vi "flushTank.vi"(8 "error in (no error)":errorcluster, 10 "Index":i32, 11 "Tank in":refnum<class "Tank.lvclass">) -> (0 "error out":errorcluster, 3 "Tank out":refnum<class "Tank.lvclass">)   [LabVIEW 2018, in "Tank.lvclass"]
uses:
  Tank.lvclass
  Tank.lvclass/Tank.ctl
  Sensor Class/Sensor.lvclass/Sensor.ctl
  Sensor Class/Sensor.lvclass
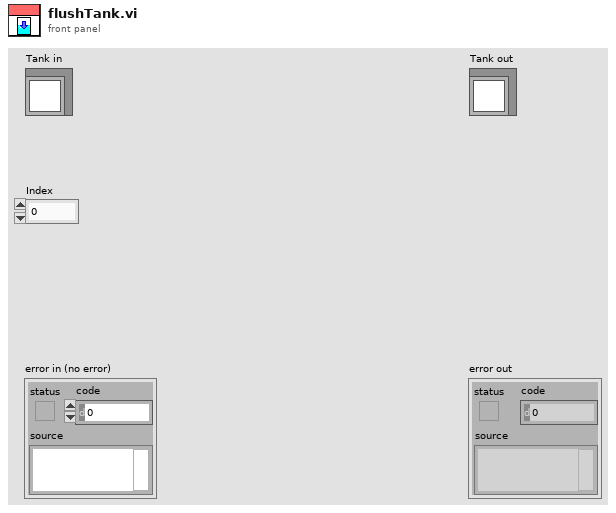
[diagram p1: front panel]
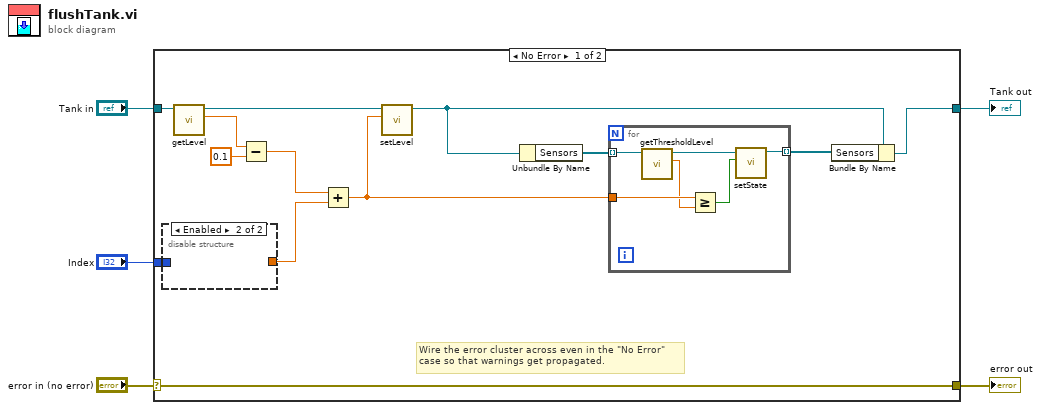
[diagram p0: block diagram]
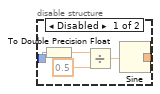
[diagram p2: hidden frame]
diagram:
  n1 = case shown="No Error" "error in (no error)" {
    selector: "error in (no error)" -> [w18 w31]
    tunnel: [w18 w31] -> w4
    tunnel: [w16 w30] -> w2
    tunnel: "Tank in" -> [w17 w30]
    tunnel: "Index" -> [w12 _]
    frame No Error {
      # "Wire the error cluster across even in the \"No Error\"\ncase so that warnings get propagated."
      n2 = disable-structure shown="Enabled" {
        disable-tunnel: [w23 _] -> w15
        disable-tunnel: w12 -> [w22 _]
        frame Disabled {
          n3 = To Double Precision Float(number=w22) -> (double precision float=w20:dbl)
          n4 = Divide(x=w20, y=0.5) -> (x/y=w21:dbl)
          n5 = Sine(x=w21) -> (sin(x)=w23:dbl)
        }
        frame Enabled {
        }
      }
      n6 = call "getLevel.vi"("Tank in"=w17) -> ("Level"=w11:dbl, "Tank out"=w9:refnum<class "Tank.lvclass">)  [unwired: 8 in, 1 out]
      n7 = Subtract(x=w11, y=0.1 ("x")) -> (x-y=w14:dbl)
      n8 = Add(x=w14, y=w15) -> (x+y=w6:dbl)
      n9 = call "setLevel.vi"("Level"=w6, "Tank in"=w9) -> ("Tank out"=w8:refnum<class "Tank.lvclass">)  [unwired: 8 in, 1 out]
      n10 = Unbundle By Name(w8) -> ("Sensors"=w10:refnum<class "Sensor.lvclass">[])
      n11 = for {
        tunnel: w10 -> [w29] mode=indexing
        tunnel: w6 -> [w25]
        tunnel: [w26] -> w7 mode=indexing
        n12 = call "getThresholdLevel.vi"("Sensor in"=w29) -> ("Threshold Level"=w24:dbl, "Sensor out"=w28:refnum<class "Sensor.lvclass">)  [unwired: 8 in, 1 out]
        n13 = Greater Or Equal?(x=w25, y=w24) -> (x >= y?=w27:bool)
        n14 = call "setState.vi"("State"=w27, "Sensor in"=w28) -> ("Sensor out"=w26:refnum<class "Sensor.lvclass">)  [unwired: 8 in, 1 out]
      }
      n15 = Bundle By Name(cluster=w8, "Sensors"=w7) -> (w16:refnum<class "Tank.lvclass">)
    }
    frame Error {
    }
  }
  "error out" <- w4
  "Tank out" <- w2
